vi "Parallel Mode Write.vi"(8 "error in":errorcluster, 10 "Parallel Mode STS":i32, 11 "Parallel Mode in":refnum<class "Parallel Mode.lvclass">) -> (0 "error out":errorcluster, 3 "Parallel Mode out":refnum<class "Parallel Mode.lvclass">)   [LabVIEW 2023, in "Parallel Mode.lvclass"]
uses:
  Parallel Mode.lvclass
  Parallel Mode.lvclass/Parallel Mode.ctl
  <vilib>/ADAS Replay HIL/Channels/Tag Wrapper/Tag Wrapper.lvlib
  <vilib>/ADAS Replay HIL/Channels/Tag Wrapper/Polymorphic/Write Channel (I32).vi
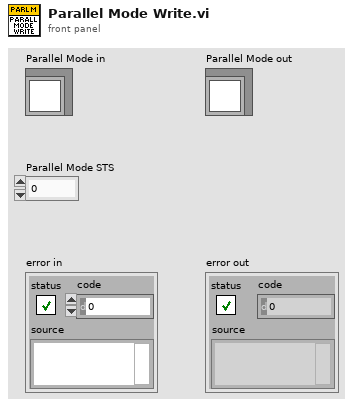
[diagram p1: front panel]
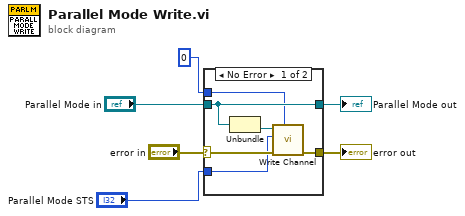
[diagram p0: block diagram]
diagram:
  n1 = case shown="No Error" "error in" {
    selector: "error in" -> [w10 w14]
    tunnel: [w9 w14] -> w5
    tunnel: [w11 w13] -> w3
    tunnel: "Parallel Mode in" -> [w11 w13]
    tunnel: "Parallel Mode STS" -> [w8 _]
    tunnel: 0 ("Timeout (ms)") -> [w7 _]
    frame No Error {
      n2 = Unbundle(w11) -> (w12:refnum<k21>)  [unwired: 1 out]
      n3 = call-poly <vilib>:"Write Channel.vi"("Timeout (ms)"=w7, "error in"=w10, "Value to Write"=w8, "ADAS HIL Channel in"=w12) -> ("error out"=w9:errorcluster)  [unwired: 5 in, 2 out]
    }
    frame Error {
    }
  }
  "error out" <- w5
  "Parallel Mode out" <- w3
